vi "Close.vi"(8 "error in (no error)":errorcluster, 11 "FunctionGenerator in":refnum<class "FunctionGenerator.lvclass">) -> (0 "error out":errorcluster, 3 "FunctionGenerator out":refnum<class "FunctionGenerator.lvclass">)   [LabVIEW 2020, in "FunctionGenerator.lvclass"]
uses:
  FunctionGenerator.lvclass
  C:/Code Projects/CircuitExplorer/AnalogDiscoveryFunction/AnalogDiscoveryFunction.lvclass
  AnalogDiscoveryFunction/AnalogDiscoveryFunction.lvclass/AnalogDiscoveryFunction.ctl
  AnalogDiscoveryFunction/GetInstrumentHandle.vi
  <vilib>/DigilentWF/DigilentWF.lvlib
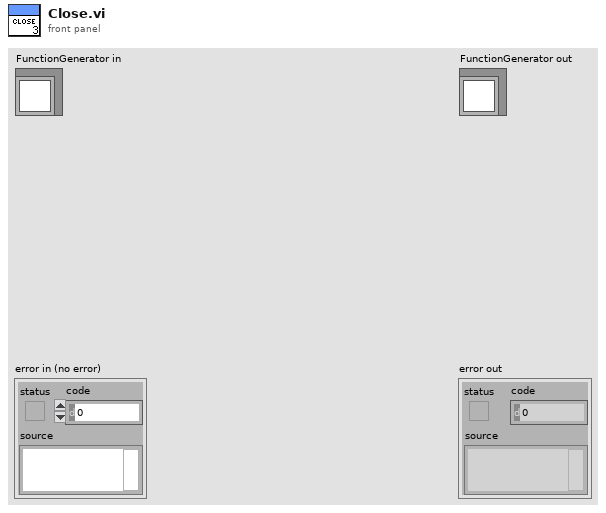
[diagram p1: front panel]
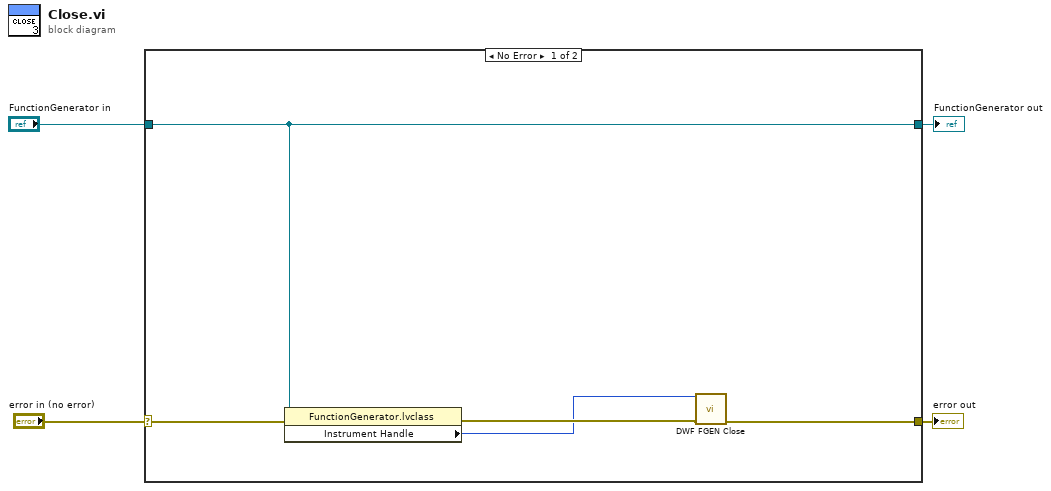
[diagram p0: block diagram]
diagram:
  n1 = case shown="No Error" "error in (no error)" {
    selector: "error in (no error)" -> [w8 w10]
    tunnel: [w6 w11] -> w2
    tunnel: "FunctionGenerator in" -> [w6 w11]
    tunnel: [w9 w10] -> w1
    frame No Error {
      n2 = property class="FunctionGenerator.lvclass"(reference=w6, error in=w8) -> (error out=w7:errorcluster, "Instrument Handle"=w5:u32)  [unwired: 1 out]
      n3 = call <vilib>:"DWF FGEN Close.vi"("Instrument Handle In"=w5, "Error In"=w7) -> ("Error Out"=w9:errorcluster)  [unwired: 13 in]
    }
    frame Error {
    }
  }
  "error out" <- w1
  "FunctionGenerator out" <- w2
